vi "Lookup Group.vi"(7 "Group Type (Abstract)":refnum<class "GroupAbstract.lvclass">, 8 "error in (no error)":errorcluster, 10 "Group Name":string, 11 "TelemetryAPI in":refnum<class "TelemetryAPI.lvclass">) -> (0 "error out":errorcluster, 2 "Group":refnum<class "GroupAbstract.lvclass">, 3 "TelemetryAPI out":refnum<class "TelemetryAPI.lvclass">)   [LabVIEW 2020, in "Volatus.lvlib" / "TelemetryAPI.lvclass"]
uses:
  TelemetryAPI.lvclass
  TelemetryAPI.lvclass/TelemetryAPI.ctl
  lv-vecto/Vecto/ChannelService/ChannelService.lvclass
  lv-vecto/Vecto/GroupAbstract/GroupAbstract.lvclass
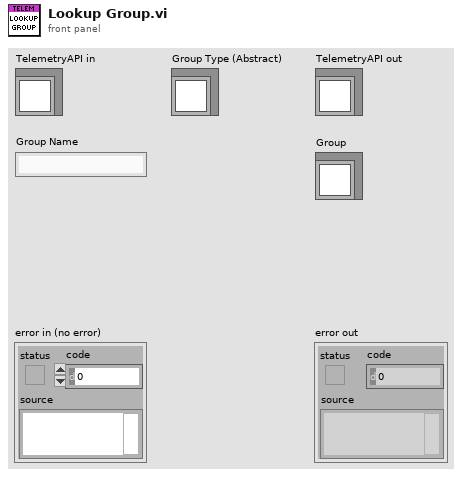
[diagram p1: front panel]
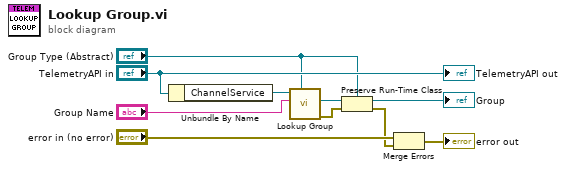
[diagram p0: block diagram]
diagram:
  n1 = Unbundle By Name("TelemetryAPI in") -> ("ChannelService"=w8:refnum<class "ChannelService.lvclass">)
  n2 = call "Lookup Group.vi"("Group Type (Abstract)"="Group Type (Abstract)", "Group Name"="Group Name", "ChannelService in"=w8) -> ("error out"=w5:errorcluster, "Group"=w7:refnum<class "GroupAbstract.lvclass">)  [unwired: 6 in, 1 out]
  n3 = Preserve Run-Time Class(object in=w7, error in=w5, 2:"Group Type (Abstract)") -> (object out=→"Group":refnum<class "GroupAbstract.lvclass">, error out=w1:errorcluster)
  n4 = Merge Errors("error in (no error)", w1) -> (→"error out":errorcluster)
  "TelemetryAPI out" <- "TelemetryAPI in"
